vi "运维调试_采配水V1.vi"() -> ()   [LabVIEW 2016, in "PLC.lvlib"]
uses:
  PLC.lvlib
  <vilib>/Plasmionique/MB Master/MB_Master/MB_Master.lvclass
  <vilib>/Utility/miscctls.llb/LVPointTypeDef.ctl
  <vilib>/Plasmionique/MB Master/MB_Master_Serial/MB_Master_Serial.lvclass
  C:/Program Files (x86)/National Instruments/LabVIEW 2016/vi.lib/Plasmionique/MB Master/MB_Master/MB_Master.lvclass
  <vilib>/Instr/_visa.llb/VISA Configure Serial Port (Instr).vi
  <vilib>/Plasmionique/MB Master/MB Master.lvlib
panel:
  out "Registers":u16[](array[numeric])
  out "R118":i16 caption="多参数沉淀时间"
  in  "更新程序":bool
  out "当前启动泵号":u16(ring) items=["1号水样泵", "2号水样泵"]
  out "R113":i16 caption="储水时间设定"
  out "X2":bool caption="X1"
  out "采配水版本号":string
  out "R23":i16 caption="清洗频次计数"
  out "R112":i16 caption="清洗频次设定"
  out "R22":i16
  in  "Y15":bool
  out "R111":i16 caption="排液时间"
  out "通讯故障":bool
  out "R21":i16
  in  "Y14":bool
  out "R20":i16
  in  "Y13":bool
  in  "潜水泵工作模式":u16(ring) items=["泵1单泵单管路", "泵2单泵单管路", "潜水泵双泵双管路", "自吸泵双泵双管路"]
  out "X10":bool caption="废液报警"
  out "X9":bool caption="自来水检测"
  out "X8":bool caption="泵2过载报警"
  out "X7":bool caption="泵1过载报警"
  out "X6":bool caption="断电检测"
  out "X5":bool caption="开门检测"
  out "X4":bool caption="烟雾检测"
  out "X3":bool caption="漏水检测"
  out "X1":bool
  out "X0":bool caption="采样池液位开关"
  out "R109":i16 caption="配水时间"
  out "集成报警信息":string
  out "R108":i16 caption="自来水报警"
  out "R107":i16 caption="采水池液位报警设置"
  out "R106":i16 caption="进样超时设置"
  out "R105":i16 caption="二级清洗时间"
  out "R104":i16 caption="一级清洗时间"
  out "R103":i16 caption="外部管路清洗时间"
  out "R102":i16 caption="静置沉淀时间"
  out "R101":i16 caption="内部管路润洗时间"
  out "R100":i16 caption="外部管路润洗时间"
  out "R2":i16
  out "R1":i16
  out "多列列表框":i32(listbox)
  out "R19":i16
  in  "Y7":bool
  out "R18":i16
  in  "Y6":bool
  out "R17":i16
  in  "Y5":bool
  out "R16":i16
  in  "Y4":bool
  out "R15":i16
  in  "Y3":bool
  out "R14":i16
  in  "Y2":bool
  out "R13":i16
  in  "Y1":bool
  out "R12":i16
  in  "Y0":bool
  in  "返回":bool
  in  "参数设置":bool
  in  "单步启动":bool
  in  "启动":bool
  in  "停止":bool
  # "S"
  # "S"
  # "次"
  # "次"
  # "S"
  # "S"
  # "S"
  # "S"
  # "S"
  # "S"
  # "S"
  # "S"
  # "S"
  # "S"
  # "S"
  # "单步计时："
  # "s"
  # "流程计时："
  # "s"
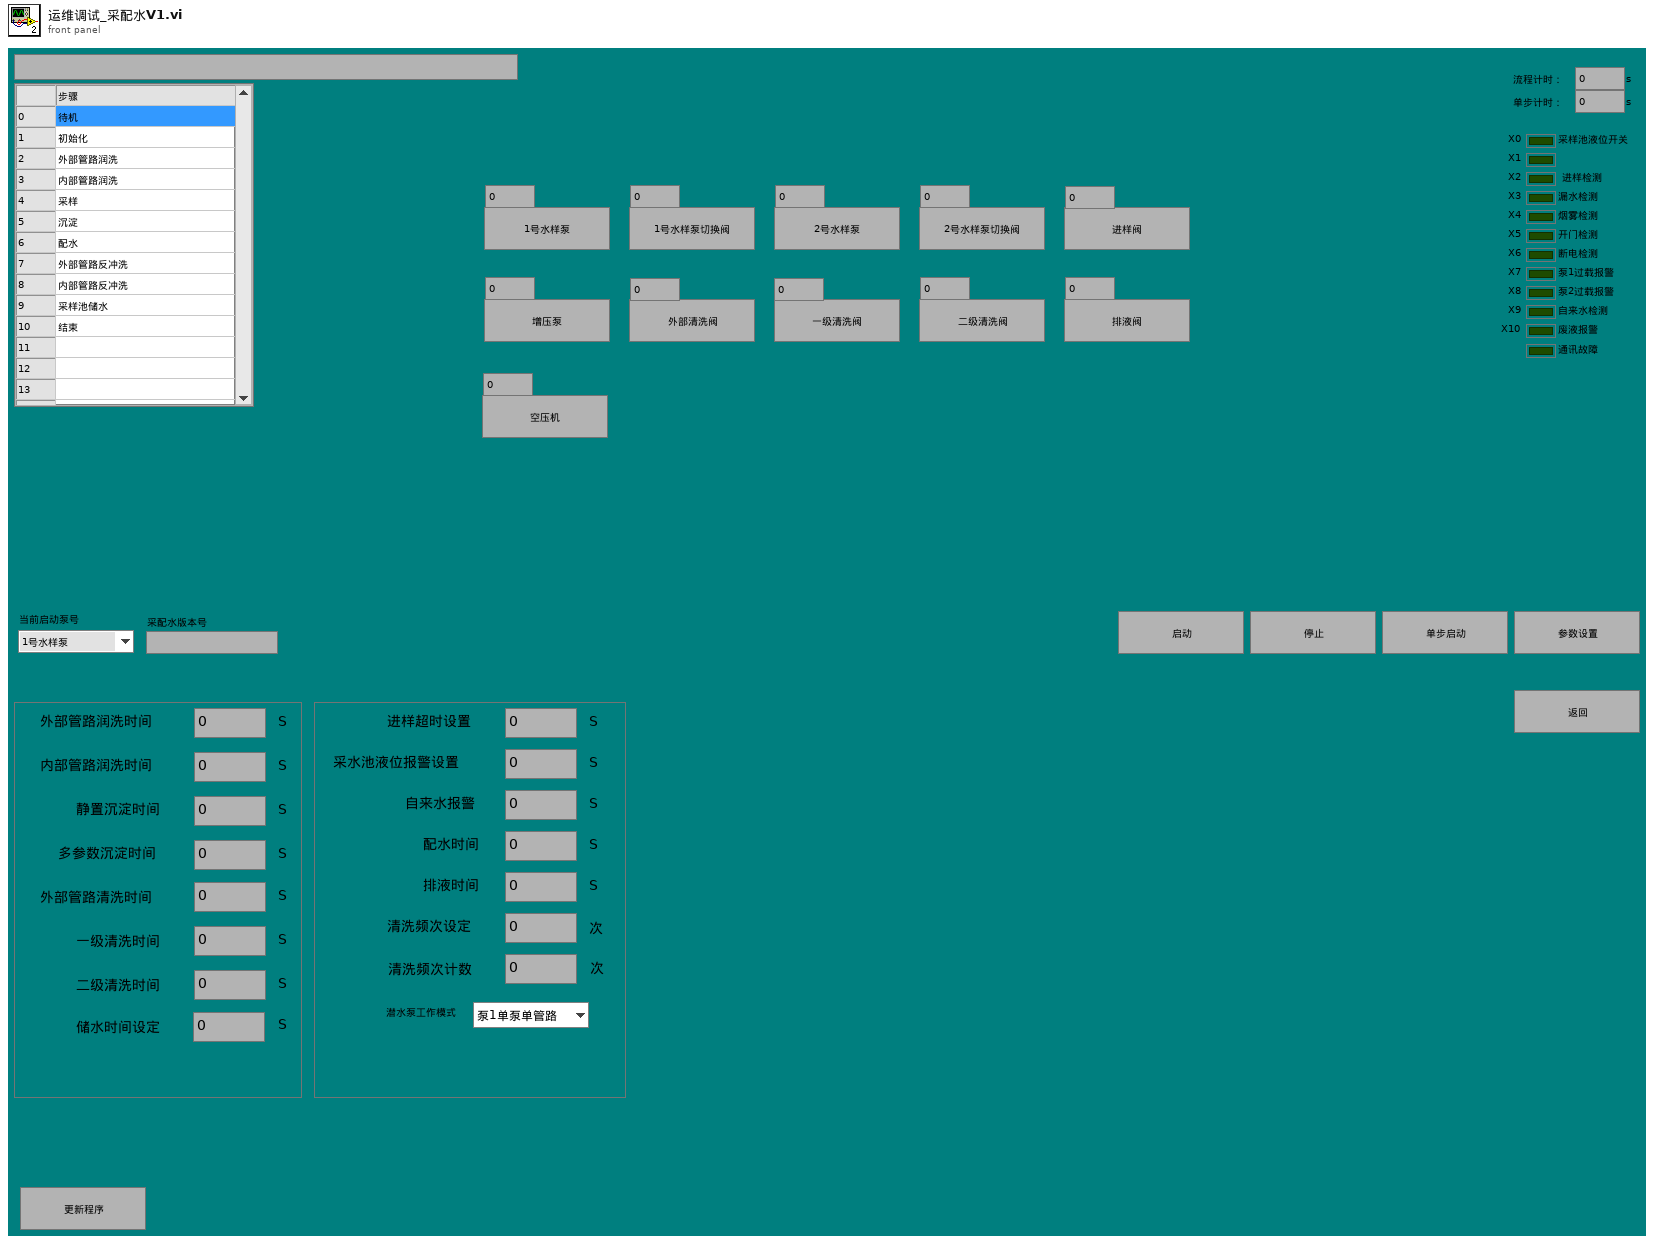
[diagram p1: front panel]
types:
  T1 = typedef "参数.ctl" = cluster{"测试模式":enum16{"水样测试", "平行样测试", "集成干预测试", "加标回收"}, "参数启用":T2}
  T2 = typedef "启动参数.ctl" = cluster{"氨氮":bool, "总磷":bool, "总氮":bool, "多参数":bool, "CODmn":bool, "CODCr":bool, "氟化物":bool, "超标留样启用":bool, "重金属":bool}
  T3 = typedef "LVPointTypeDef.ctl" = cluster{"Horizontal":i16, "Vertical":i16}
  T4 = cluster{"命令":string, "数据":cluster{"starting address":u16, "holding register value":u16}}
  T5 = cluster{"R0":i16, "R1":i16, "R2":i16, "R3":i16, "R4":i16, "R5":i16, "R6":i16, "R7":i16, "R8":i16, "R9":i16, "R10":i16, "R11":i16, "R12":i16, "R13":i16, "R14":i16, "R15":i16, "R16":i16, "R17":i16, "R18":i16, "R19":i16, "R20":i16, "R21":i16, "R22":i16, "R23":i16, "R24":i16, "R25":i16, "R26":i16, "R27":i16, "R28":i16, "R29":i16, "R30":i16, "R31":i16, "R32":i16, "R33":i16, "R34":i16, "R35":i16, "R36":i16, "R37":i16, "R38":i16, "R39":i16, "R40":i16, "R41":i16, "R42":i16, "R43":i16, "R44":i16, "R45":i16, "R46":i16, "R47":i16, "R48":i16, "R49":i16, "R50":i16, "R51":i16, "R52":i16, "R53":i16, "R54":i16, "R55":i16, "R56":i16, "R57":i16, "R58":i16, "R59":i16, "R60":i16, "R61":i16, "R62":i16, "R63":i16, "R64":i16, "R65":i16, "R66":i16, "R67":i16, "R68":i16, "R69":i16, "R70":i16, "R71":i16, "R72":i16, "R73":i16, "R74":i16, "R75":i16, "R76":i16, "R77":i16, "R78":i16, "R79":i16}
  T6 = cluster{"seconds since 1Jan1904":timestamp, "table输入":string, string, "table输入":string}
  T7 = cluster{"命令":string, cluster{"starting address":u16, "holding register value":u16}}
  T8 = cluster{"命令":string, "数据":cluster{"starting address":u16, "holding register values":u16[]}}
  T9 = cluster{"命令":string, "data":cluster{"starting address":u16, "coil values":bool[]}}
  T10 = cluster{"测试模式":enum16{"水样测试", "平行样测试", "集成干预测试", "加标回收"}, "参数启用":T2}
  T11 = cluster{"baud rate (bps)":u32, "stop bits":u16, "parity":u16, "flow control":u16, "timeout":u32, "retries":i32}
  T12 = cluster{"starting address":u16, "holding register values":u16[]}
  T13 = cluster{"starting address":u16, "holding register value":u16}
  T14 = cluster{"starting address":u16, "coil values":bool[]}
  T15 = cluster{"Registers[0]":u16, "Registers[1]":u16, "Registers[2]":u16, "Registers[3]":u16, "Registers[4]":u16, "Registers[5]":u16, "Registers[6]":u16, "Registers[7]":u16, "Registers[8]":u16, "Registers[9]":u16, "Registers[10]":u16, "Registers[11]":u16, "Registers[12]":u16, "Registers[13]":u16, "Registers[14]":u16, "Registers[15]":u16, "Registers[16]":u16, "Registers[17]":u16, "Registers[18]":u16, "Registers[19]":u16, "Registers[20]":u16, "Registers[21]":u16, "Registers[22]":u16, "Registers[23]":u16, "Registers[24]":u16, "Registers[25]":u16, "Registers[26]":u16, "Registers[27]":u16, "Registers[28]":u16, "Registers[29]":u16, "Registers[30]":u16, "Registers[31]":u16, "Registers[32]":u16, "Registers[33]":u16, "Registers[34]":u16, "Registers[35]":u16, "Registers[36]":u16, "Registers[37]":u16, "Registers[38]":u16, "Registers[39]":u16, "Registers[40]":u16, "Registers[41]":u16, "Registers[42]":u16, "Registers[43]":u16, "Registers[44]":u16, "Registers[45]":u16, "Registers[46]":u16, "Registers[47]":u16, "Registers[48]":u16, "Registers[49]":u16, "Registers[50]":u16, "Registers[51]":u16, "Registers[52]":u16, "Registers[53]":u16, "Registers[54]":u16, "Registers[55]":u16, "Registers[56]":u16, "Registers[57]":u16, "Registers[58]":u16, "Registers[59]":u16, "Registers[60]":u16, "Registers[61]":u16, "Registers[62]":u16, "Registers[63]":u16, "Registers[64]":u16, "Registers[65]":u16, "Registers[66]":u16, "Registers[67]":u16, "Registers[68]":u16, "Registers[69]":u16, "Registers[70]":u16, "Registers[71]":u16, "Registers[72]":u16, "Registers[73]":u16, "Registers[74]":u16, "Registers[75]":u16, "Registers[76]":u16, "Registers[77]":u16, "Registers[78]":u16, "Registers[79]":u16}
  T16 = cluster{"Registers[0]":u16, "Registers[1]":u16, "Registers[2]":u16, "Registers[3]":u16, "Registers[4]":u16, "Registers[5]":u16}
  T17 = cluster{"Registers[0]":u16, "Registers[1]":u16, "Registers[2]":u16, "Registers[3]":u16, "Registers[4]":u16, "Registers[5]":u16, "Registers[6]":u16, "Registers[7]":u16, "Registers[8]":u16, "Registers[9]":u16, "Registers[10]":u16, "Registers[11]":u16, "Registers[12]":u16, "Registers[13]":u16, "Registers[14]":u16, "Registers[15]":u16, "Registers[16]":u16, "Registers[17]":u16, "Registers[18]":u16, "Registers[19]":u16, "Registers[20]":u16, "Registers[21]":u16, "Registers[22]":u16, "Registers[23]":u16, "Registers[24]":u16, "Registers[25]":u16, "Registers[26]":u16, "Registers[27]":u16, "Registers[28]":u16, "Registers[29]":u16, "Registers[30]":u16, "Registers[31]":u16, "Registers[32]":u16, "Registers[33]":u16}
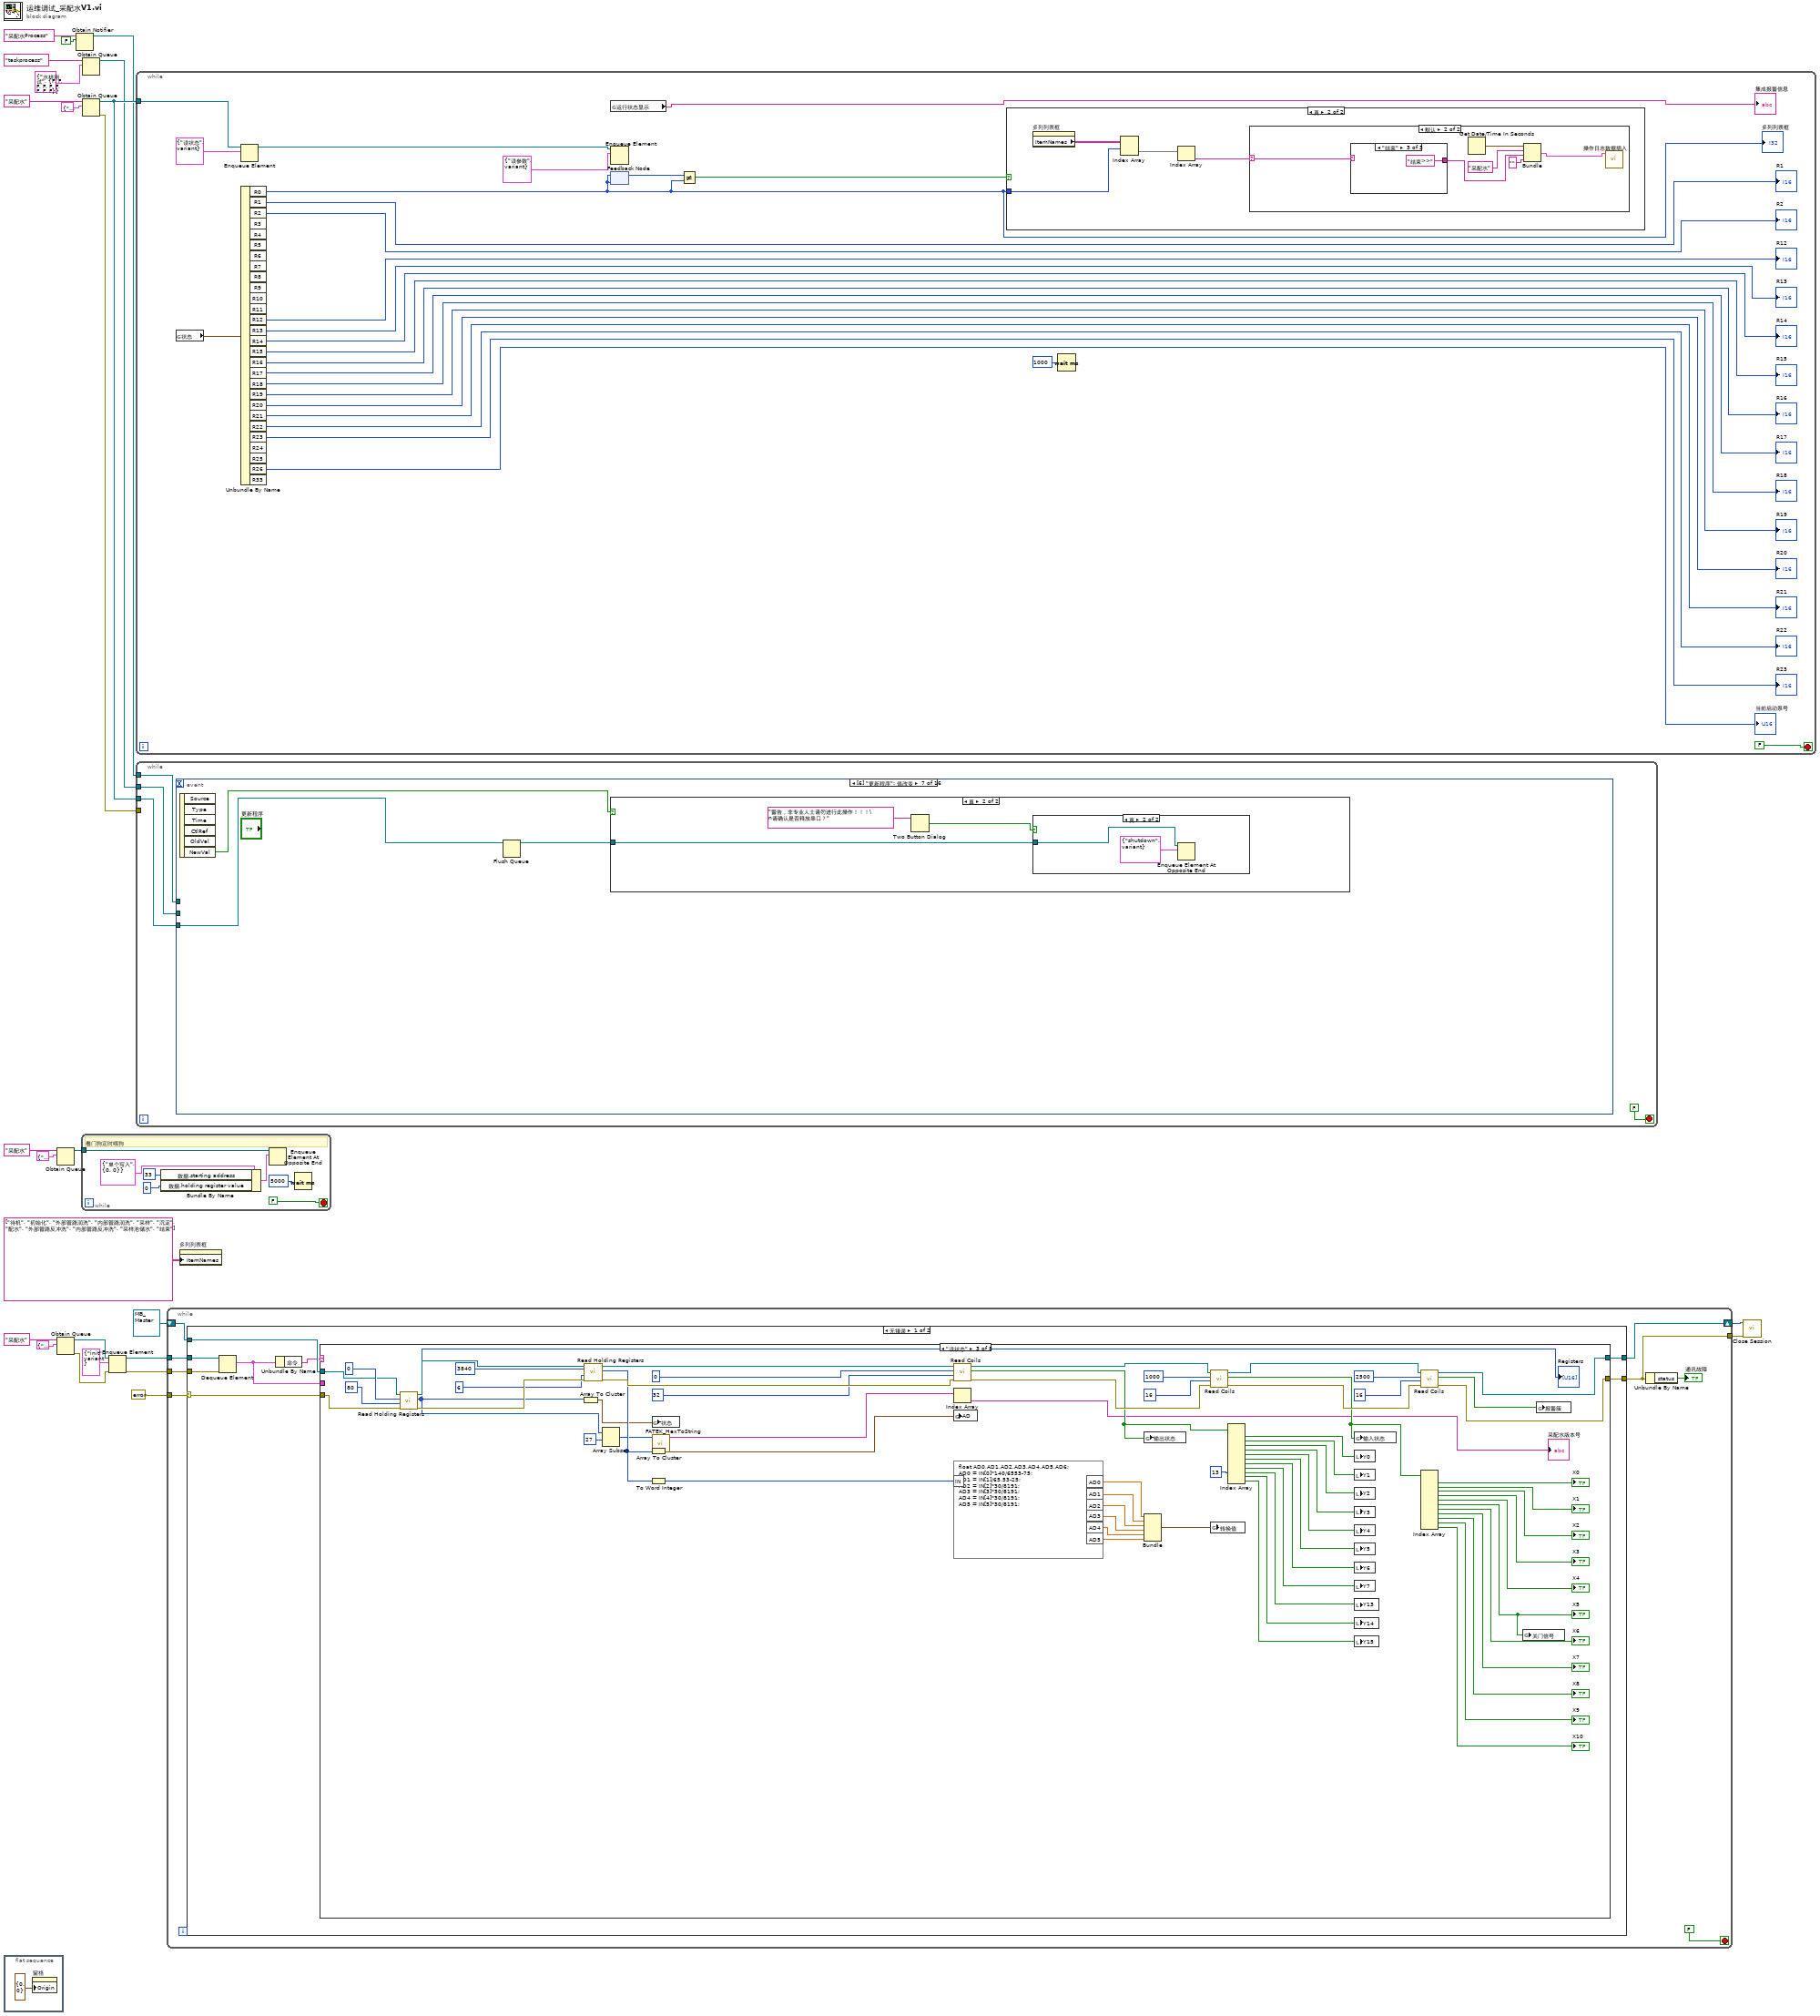
[diagram p0: block diagram]
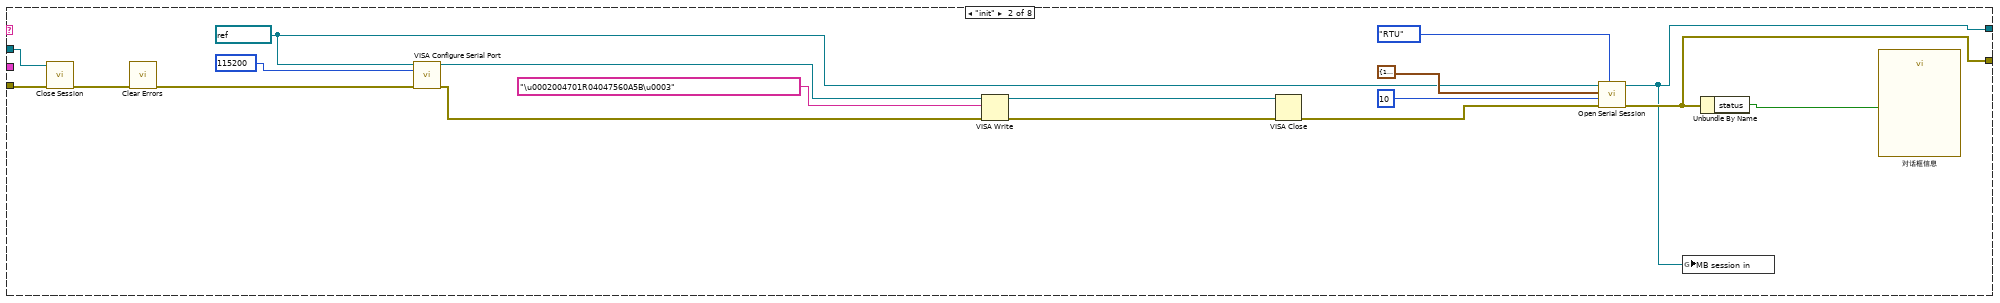
[diagram p3: hidden frame]
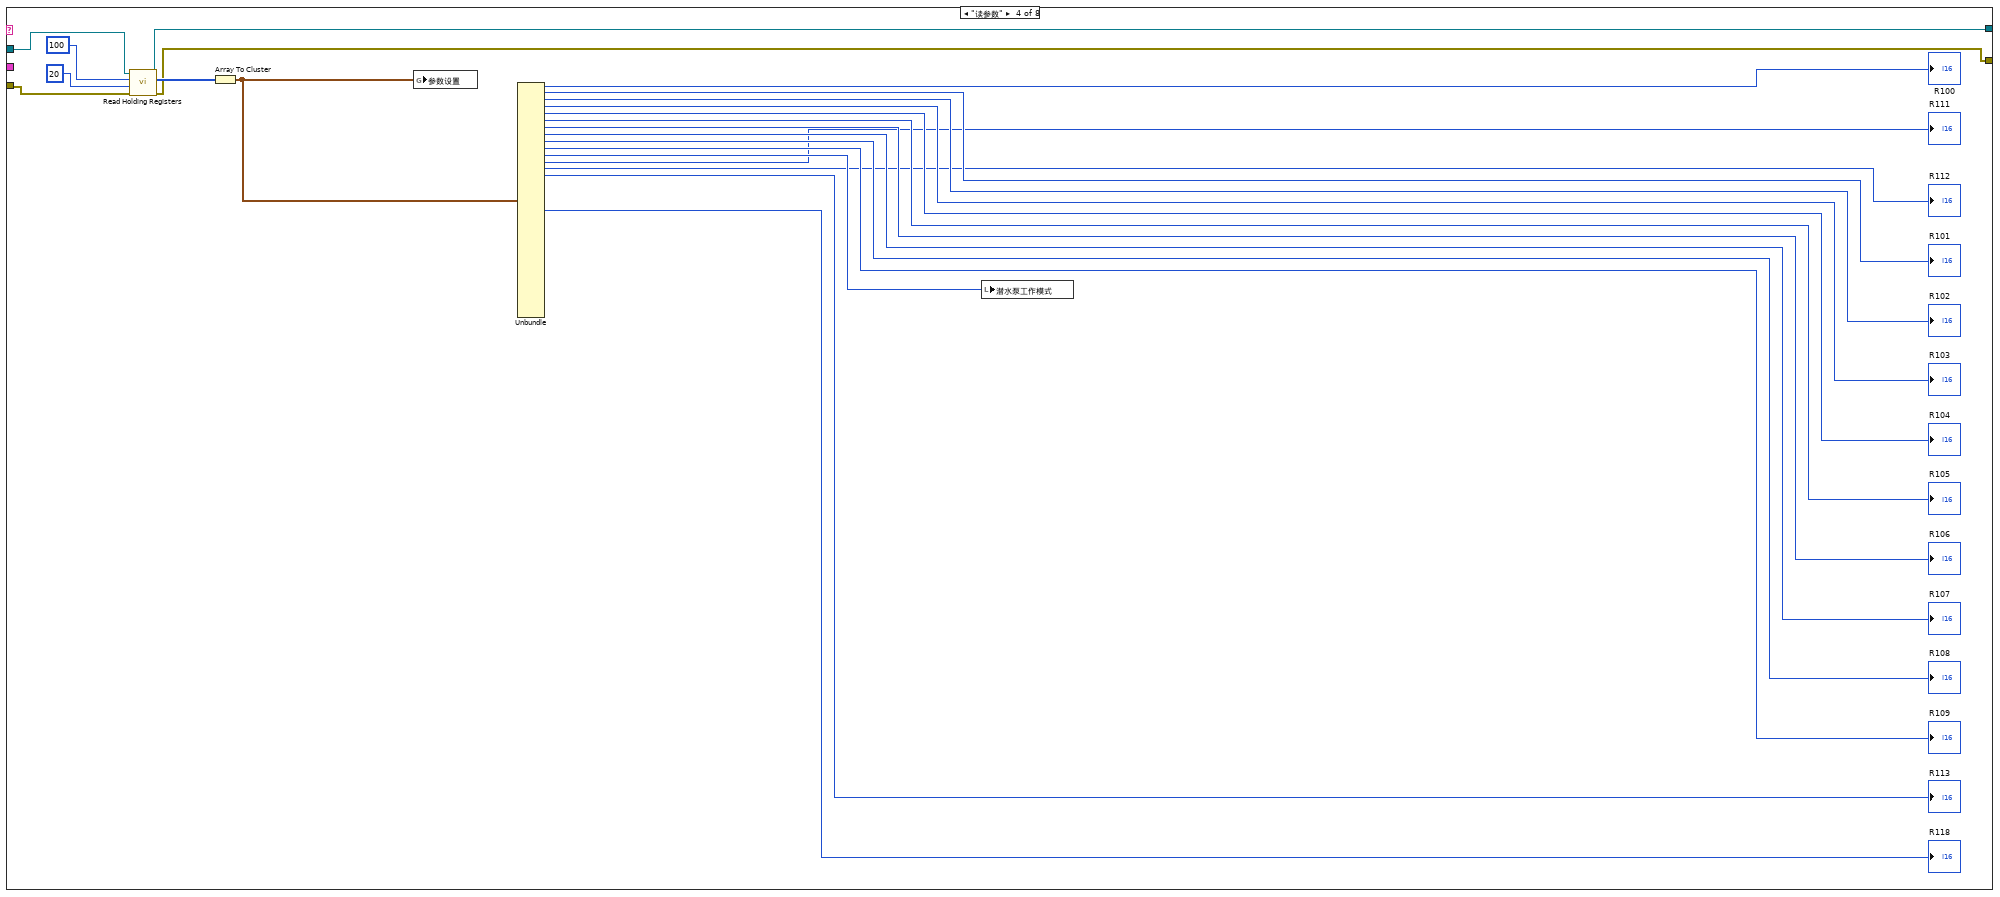
[diagram p4: hidden frame]
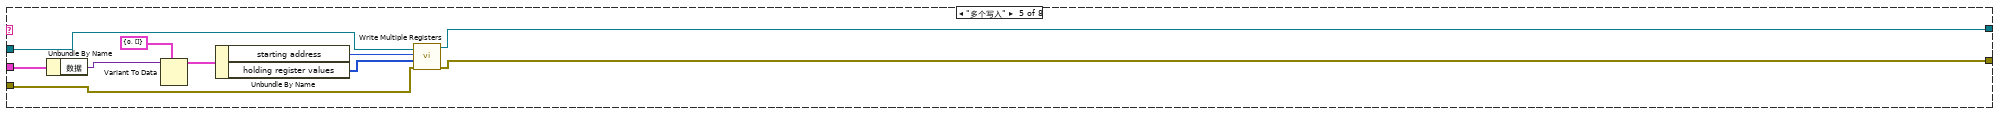
[diagram p5: hidden frame]
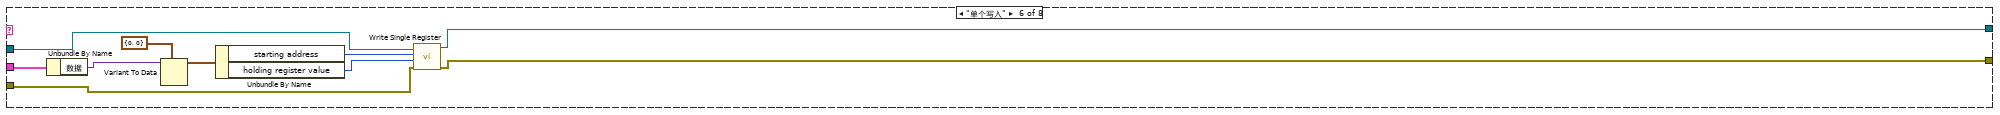
[diagram p6: hidden frame]
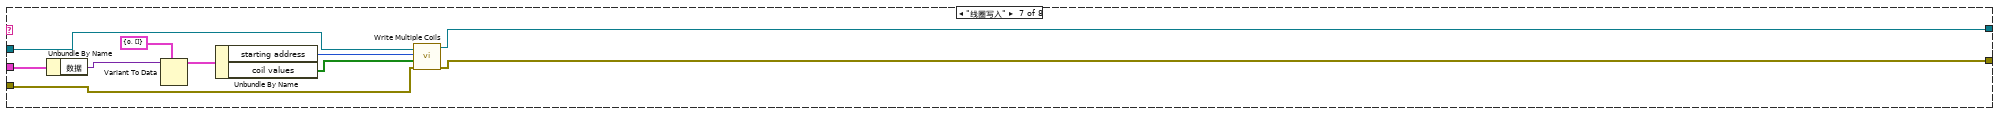
[diagram p7: hidden frame]
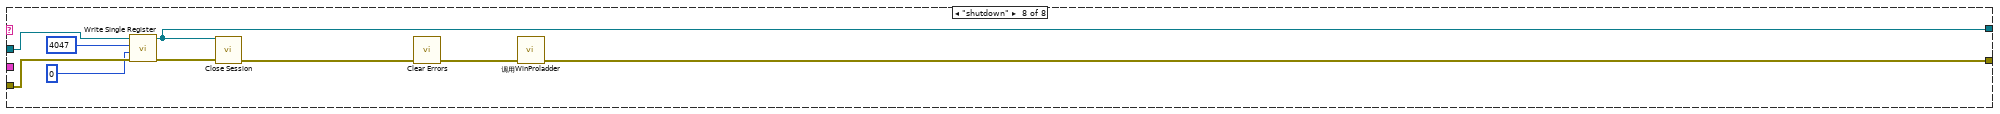
[diagram p8: hidden frame]
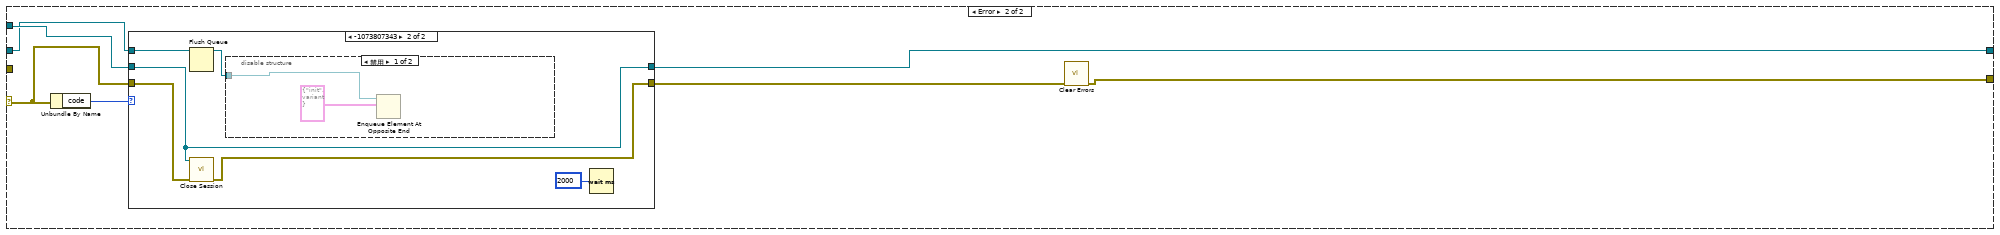
[diagram p9: hidden frame]
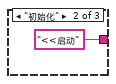
[diagram p15: hidden frame]
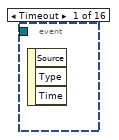
[diagram p16: hidden frame]
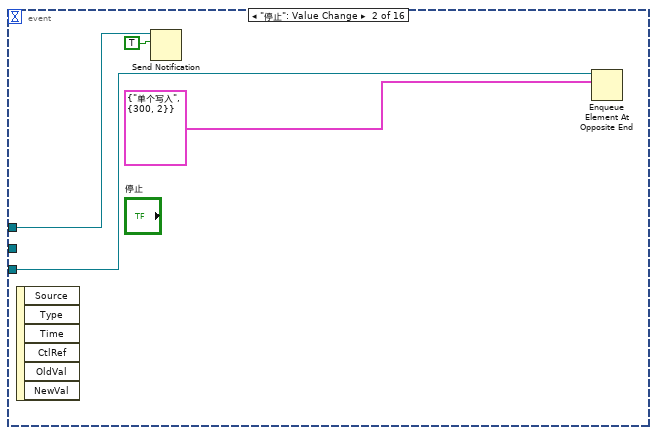
[diagram p17: hidden frame]
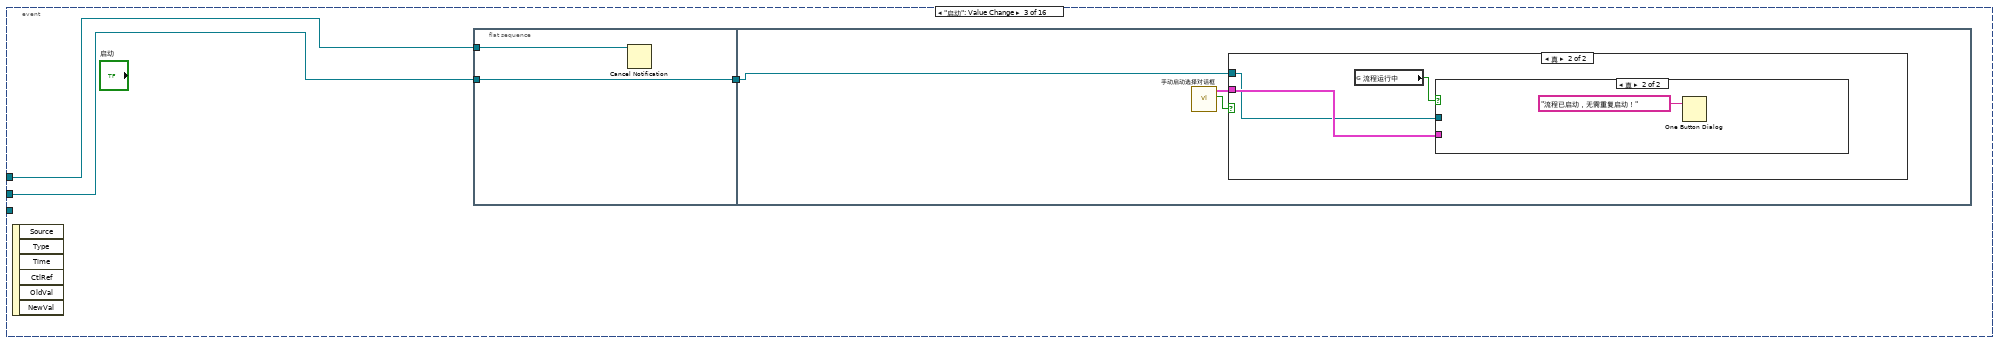
[diagram p18: hidden frame]
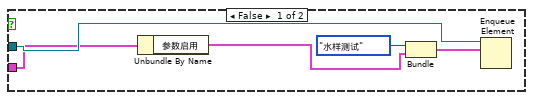
[diagram p20: hidden frame]
diagram:
  n1 = flat-sequence {
    frame #0 {
      n2 = property on="窗格" class="Pane"("Origin"=T3 {"Horizontal"=0, "Vertical"=0} ("原点")) -> ()  [unwired: 2 in, 2 out]
    }
  }
  n3 = Obtain Queue(name (unnamed)="采配水" ("名称（未命名）"), element data type=cluster{"命令":string, "数据":variant} {"命令"="", "数据"=variant}) -> (queue out=w4:refnum<queue>)  [unwired: 3 in, 2 out]
  n4 = Obtain Queue(name (unnamed)="采配水" ("名称（未命名）"), element data type=cluster{"命令":string, "数据":variant} {"命令"="", "数据"=variant}) -> (queue out=w15:refnum<queue>, error out=w14:errorcluster)  [unwired: 3 in, 1 out]
  n5 = Obtain Notifier(name (unnamed)="采配水Process" ("名称（未命名）"), notification data type=FALSE) -> (notifier out=w18:refnum<notifier>)  [unwired: 2 in, 2 out]
  n6 = while {
    tunnel: w4 -> [w29]
    stop <- FALSE stop-if-true
    # "看门狗定时喂狗"
    n7 = Bundle By Name(cluster=T4 {"命令"="单个写入", "数据"={"starting address"=0, "holding register value"=0}} ("元素"), "数据.starting address"=u16 33, "数据.holding register value"=u16 0) -> (w30:T4)
    n8 = Enqueue Element At Opposite End(queue=w29, element=w30) -> ()  [unwired: 2 in, 3 out]
    n9 = Wait (ms)(milliseconds to wait=u32 5000 ("等待时间（毫秒）")) -> ()  [unwired: 1 out]
  }
  n10 = Obtain Queue(name (unnamed)="taskprocess" ("名称（未命名）"), element data type=T1 {"测试模式"=enum."水样测试", "参数启用"={"氨氮"=FALSE, "总磷"=FALSE, "总氮"=FALSE, "多参数"=FALSE, "CODmn"=FALSE, "CODCr"=FALSE, "氟化物"=FALSE, "超标留样启用"=FALSE, "重金属"=FALSE}} ("参数")) -> (queue out=w2:refnum<queue>)  [unwired: 3 in, 2 out]
  n11 = Obtain Queue(name (unnamed)="采配水" ("名称（未命名）"), element data type=cluster{"命令":string, "数据":variant} {"命令"="", "数据"=variant}) -> (queue out=w22:refnum<queue>, error out=w23:errorcluster)  [unwired: 3 in, 1 out]
  n12 = Enqueue Element(queue=w15, element=cluster{"命令":string, "数据":variant} {"命令"="init", "数据"=variant} ("元素"), error in (no error)=w14) -> (queue out=w10:refnum<queue>, error out=w12:errorcluster)  [unwired: 1 in, 1 out]
  n13 = while {
    tunnel: w22 -> [w58]
    stop <- FALSE stop-if-true
    n14 = global read "采配水全局变量.vi" "状态"() -> (w56:T5)
    n15 = Enqueue Element(queue=w58, element=cluster{"命令":string, "数据":variant} {"命令"="读状态", "数据"=variant} ("元素")) -> (queue out=w41:refnum<queue>)  [unwired: 2 in, 2 out]
    n16 = Unbundle By Name(w56) -> ("R0"=w39:i16, "R1"=→"R1":i16, "R2"=→"R2":i16, "R12"=→"R12":i16, "R13"=→"R13":i16, "R14"=→"R14":i16, "R15"=→"R15":i16, "R16"=→"R16":i16, "R17"=→"R17":i16, "R18"=→"R18":i16, "R19"=→"R19":i16, "R20"=→"R20":i16, "R21"=→"R21":i16, "R22"=→"R22":i16, "R23"=→"R23":i16, "R26"=→"当前启动泵号":i16)  [unwired: 12 out]
    "多列列表框" <- w39
    n17 = global read "采配水全局变量.vi" "运行状态显示"() -> (→"集成报警信息":string)
    n18 = Enqueue Element(queue=w41, element=cluster{"命令":string, "数据":variant} {"命令"="读参数", "数据"=variant} ("元素")) -> ()  [unwired: 2 in, 3 out]
    n19 = feedback-in #1(w39) -> ()
    n20 = feedback #1(w39) -> (w40:i16)
    n21 = Not Equal?(x=w40, y=w39) -> (x != y?=w45:bool)
    n22 = case shown="真" w45 {
      tunnel: w39 -> [_ w62]
      frame False {
      }
      frame True {
        n23 = property on="多列列表框" class="MCListbox (严格)"() -> ("ItemNames"=w63:string[][])  [unwired: 2 in, 2 out]
        n24 = Index Array(array=w63, index (row)=w62) -> (element=w61:string[])  [unwired: 1 in]
        n25 = Index Array(array=w61) -> (element=w60:string)  [unwired: 1 in]
        n26 = case shown="默认" w60 {
          selector: w60 -> [_ w64]
          frame "待机" {
          }
          frame Default {
            n27 = case shown="\"结束\"" w64 {
              selector: w64 -> [w70 _ _]
              tunnel: [w70 "<<启动" "结束>>"] -> w66
              frame Default {
              }
              frame "初始化" {
              }
              frame "结束" {
              }
            }
            n28 = Get Date/Time In Seconds() -> (seconds since 1Jan1904=w69:timestamp)
            n29 = Bundle("seconds since 1Jan1904"=w69, "table输入"="采配水", w66, "table输入"="") -> (w65:T6)  [unwired: 1 in]
            n30 = call "操作日志数据插入.vi"("data"=w65) -> ()  [unwired: 9 in, 1 out]
          }
        }
      }
    }
    n31 = Wait (ms)(milliseconds to wait=u32 1000 ("等待时间（毫秒）")) -> ()  [unwired: 1 out]
  }
  n32 = while {
    tunnel: w22 -> [w75]
    tunnel: w23 -> [_]
    tunnel: w18 -> [w74]
    tunnel: w2 -> [w73]
    stop <- FALSE stop-if-true
    n33 = event shown="[6] \"更新程序\": 值改变" {
      selector: _ -> [_ _ _ _ _ _ _ _ _ _ _ _ _ _ _ _]
      dyn-events: _ -> [_ _ _ _ _ _ _ _ _ _ _ _ _ _ _ _]
      timeout: _ -> [_ _ _ _ _ _ _ _ _ _ _ _ _ _ _ _]
      tunnel: w75 -> [_ w79 _ w101 w120 w123 w129 w140 _ _ _ _ w168 w170 w175 w180]
      tunnel: w74 -> [_ w78 w83 _ _ _ _ _ _ _ _ _ _ _ _ _]
      tunnel: w73 -> [_ _ w81 _ _ _ _ _ _ _ _ _ _ _ _ _]
      event Timeout {
        n34 = event-data() -> ()  [unwired: 1 in, 3 out]
      }
      event "停止": Value Change {
        n35 = event-data() -> ()  [unwired: 1 in, 6 out]
        n36 = Send Notification(notification=TRUE ("通知"), notifier=w78) -> ()  [unwired: 1 in, 2 out]
        n37 = Enqueue Element At Opposite End(queue=w79, element=T7 {"命令"="单个写入", {"starting address"=300, "holding register value"=2}} ("元素")) -> ()  [unwired: 2 in, 3 out]
      }
      event "启动": Value Change {
        n38 = event-data() -> ()  [unwired: 1 in, 6 out]
        n39 = flat-sequence {
          tunnel: w83 -> [w85]
          tunnel: [w84] -> w82
          tunnel: w81 -> [w84]
          tunnel: w82 -> [w86]
          frame #0 {
            n40 = Cancel Notification(0:w85) -> ()  [unwired: 1 in, 3 out]
          }
          frame #1 {
            n41 = call "手动启动选择对话框.vi"() -> ("确定"=w87:bool, "输出簇"=w88:cluster{"参数启用":T2})  [unwired: 10 in]
            n42 = case shown="真" w87 {
              tunnel: w88 -> [_ w91]
              tunnel: w86 -> [_ w90]
              frame False {
              }
              frame True {
                n43 = global read "采配水全局变量.vi" "流程运行中"() -> (w89:bool)
                n44 = case shown="真" w89 {
                  tunnel: w91 -> [w94 _]
                  tunnel: w90 -> [w96 _]
                  frame False {
                    n45 = Unbundle By Name(w94) -> ("参数启用"=w93:T2)
                    n46 = Bundle("测试模式"=enum16{"水样测试", "平行样测试", "集成干预测试", "加标回收"}."水样测试", "参数启用"=w93) -> (w92:T10)  [unwired: 1 in]
                    n47 = Enqueue Element(queue=w96, element=w92) -> ()  [unwired: 2 in, 3 out]
                  }
                  frame True {
                    n48 = One Button Dialog(message="流程已启动，无需重复启动！" ("消息")) -> ()  [unwired: 1 in, 1 out]
                  }
                }
              }
            }
          }
        }
      }
      event "单步启动": Value Change {
        n49 = event-data() -> ()  [unwired: 1 in, 6 out]
        n50 = call "单步启动对话框.vi"() -> ("单步启动步骤输出"=w98:u16)  [unwired: 11 in]
        n51 = Bundle By Name(cluster=T4 {"命令"="单个写入", "数据"={"starting address"=301, "holding register value"=0}} ("元素"), "数据.holding register value"=w98) -> (w99:T4)
        n52 = Enqueue Element At Opposite End(queue=w101, element=w99) -> ()  [unwired: 2 in, 3 out]
      }
      event "R100", "R101", "R102", "R103", "R104", "R105", "R106", "R107", "R108", "R109", "潜水泵工作模式", "R111", "R112", "R113": Value Change {
        n53 = event-data() -> ()  [unwired: 1 in, 6 out]
        n54 = local read "R100"() -> (w115:i16)
        n55 = local read "R101"() -> (w114:i16)
        n56 = local read "R102"() -> (w113:i16)
        n57 = local read "R103"() -> (w112:i16)
        n58 = local read "R104"() -> (w111:i16)
        n59 = local read "R105"() -> (w110:i16)
        n60 = local read "R106"() -> (w109:i16)
        n61 = local read "R107"() -> (w108:i16)
        n62 = local read "R108"() -> (w107:i16)
        n63 = local read "R109"() -> (w106:i16)
        n64 = local read "R111"() -> (w104:i16)
        n65 = local read "R112"() -> (w103:i16)
        n66 = local read "R113"() -> (w102:i16)
        n67 = Build Array(w115, w114, w113, w112, w111, w110, w109, w108, w107, w106, "潜水泵工作模式", w104, w103, w102) -> (w116:u16[])
        n68 = Bundle By Name(cluster=T8 {"命令"="多个写入", "数据"={"starting address"=0, "holding register values"=[]}} ("元素"), "数据.starting address"=u16 100, "数据.holding register values"=w116) -> (w117:T8)
        n69 = Enqueue Element At Opposite End(queue=w120, element=w117) -> ()  [unwired: 2 in, 3 out]
      }
      event "R118": Value Change {
        n70 = event-data() -> ()  [unwired: 1 in, 6 out]
        n71 = local read "R118"() -> (w121:i16)
        n72 = Build Array(w121) -> (w122:i16[])
        n73 = Bundle By Name(cluster=T8 {"命令"="多个写入", "数据"={"starting address"=0, "holding register values"=[]}} ("元素"), "数据.starting address"=u16 118, "数据.holding register values"=w122) -> (w124:T8)
        n74 = Enqueue Element At Opposite End(queue=w123, element=w124) -> ()  [unwired: 2 in, 3 out]
      }
      event "更新程序": Value Change {
        n75 = event-data() -> ("NewVal"=w128:bool)  [unwired: 1 in, 5 out]
        n76 = Flush Queue(queue=w129) -> (queue out=w127:refnum<queue>)  [unwired: 1 in, 2 out]
        n77 = case shown="真" w128 {
          tunnel: w127 -> [w130 w134]
          frame False {
            n78 = Enqueue Element At Opposite End(queue=w130, element=cluster{"命令":string, "数据":variant} {"命令"="init", "数据"=variant} ("元素")) -> ()  [unwired: 2 in, 3 out]
          }
          frame True {
            n79 = Two Button Dialog(message="警告，非专业人士请勿进行此操作！！！\n请确认是否释放串口？" ("消息")) -> (T button?=w132:bool)  [unwired: 2 in]
            n80 = case shown="真" w132 {
              tunnel: w134 -> [_ w137]
              frame False {
                n81 = local write "更新程序"(FALSE ("下载模式")) -> ()
              }
              frame True {
                n82 = Enqueue Element At Opposite End(queue=w137, element=cluster{"命令":string, "数据":variant} {"命令"="shutdown", "数据"=variant} ("元素")) -> ()  [unwired: 2 in, 3 out]
              }
            }
          }
        }
      }
      event "R23": Value Change {
        n83 = event-data() -> ()  [unwired: 1 in, 6 out]
        n84 = local read "R23"() -> (w139:i16)
        n85 = Build Array(w139) -> (w138:i16[])
        n86 = Bundle By Name(cluster=T8 {"命令"="多个写入", "数据"={"starting address"=0, "holding register values"=[]}} ("元素"), "数据.starting address"=u16 23, "数据.holding register values"=w138) -> (w141:T8)
        n87 = Enqueue Element At Opposite End(queue=w140, element=w141) -> ()  [unwired: 2 in, 3 out]
      }
      event "R23": Mouse Down {
        n88 = event-data() -> ("CtlRef"=w146:refnum<vi>)  [unwired: 1 in, 7 out]
        n89 = Two Button Dialog(message="请确认是否更改，更改后将影响实际清洗频次" ("消息")) -> (T button?=w145:bool)  [unwired: 2 in]
        n90 = case shown="真" w145 {
          tunnel: w146 -> [_ w147]
          frame False {
          }
          frame True {
            n91 = property class="DigNum (严格)"(reference=w147) -> (reference out=w149:refnum<vi>, "Value"=w150:i16)  [unwired: 1 in, 1 out]
            n92 = call "数字键盘.vi"("OldNumber"=w150) -> ("NewNumber"=w148:sgl)
            n93 = property class="DigNum (严格)"(reference=w149, "Val(Sgnl)"=w148) -> ()  [unwired: 1 in, 2 out]
          }
        }
      }
      event "R100", "R101", "R102", "R103", "R104", "R105", "R106", "R107", "R108", "R109", "R111", "R112", "R113", "R118": Mouse Down {
        n94 = event-data() -> ("CtlRef"=w154:refnum<vi>)  [unwired: 1 in, 7 out]
        n95 = property class="DigNum (严格)"(reference=w154) -> (reference out=w152:refnum<vi>, "Value"=w153:i16)  [unwired: 1 in, 1 out]
        n96 = call "数字键盘.vi"("OldNumber"=w153) -> ("NewNumber"=w151:sgl)
        n97 = property class="DigNum (严格)"(reference=w152, "Val(Sgnl)"=w151) -> ()  [unwired: 1 in, 2 out]
      }
      event "参数设置": Value Change {
        n98 = event-data() -> ()  [unwired: 1 in, 6 out]
        n99 = property on="窗格" class="Pane"("Origin"=T3 {"Horizontal"=0, "Vertical"=628} ("原点")) -> ()  [unwired: 2 in, 2 out]
      }
      event "返回": Value Change {
        n100 = event-data() -> ()  [unwired: 1 in, 6 out]
        n101 = property on="窗格" class="Pane"("Origin"=T3 {"Horizontal"=0, "Vertical"=0} ("原点")) -> ()  [unwired: 2 in, 2 out]
      }
      event "Y0", "Y1", "Y2", "Y3", "Y4", "Y5", "Y6", "Y7": Value Change {
        n102 = event-data() -> ()  [unwired: 1 in, 6 out]
        n103 = Build Array("Y0", "Y1", "Y2", "Y3", "Y4", "Y5", "Y6", "Y7") -> (w157:bool[])
        n104 = Bundle By Name(cluster=T9 {"命令"="线圈写入", "data"={"starting address"=2400, "coil values"=[]}} ("元素"), "data.coil values"=w157) -> (w158:T9)
        n105 = Enqueue Element(queue=w168, element=w158) -> ()  [unwired: 2 in, 3 out]
      }
      event "Y13": Value Change {
        n106 = event-data() -> ()  [unwired: 1 in, 6 out]
        n107 = Build Array("Y13") -> (w171:bool[])
        n108 = Bundle By Name(cluster=T9 {"命令"="线圈写入", "data"={"starting address"=2413, "coil values"=[]}} ("元素"), "data.coil values"=w171) -> (w172:T9)
        n109 = Enqueue Element(queue=w170, element=w172) -> ()  [unwired: 2 in, 3 out]
      }
      event "Y14": Value Change {
        n110 = event-data() -> ()  [unwired: 1 in, 6 out]
        n111 = Build Array("Y14") -> (w176:bool[])
        n112 = Bundle By Name(cluster=T9 {"命令"="线圈写入", "data"={"starting address"=2414, "coil values"=[]}} ("元素"), "data.coil values"=w176) -> (w177:T9)
        n113 = Enqueue Element(queue=w175, element=w177) -> ()  [unwired: 2 in, 3 out]
      }
      event "Y15": Value Change {
        n114 = event-data() -> ()  [unwired: 1 in, 6 out]
        n115 = Build Array("Y15") -> (w181:bool[])
        n116 = Bundle By Name(cluster=T9 {"命令"="线圈写入", "data"={"starting address"=2415, "coil values"=[]}} ("元素"), "data.coil values"=w181) -> (w182:T9)
        n117 = Enqueue Element(queue=w180, element=w182) -> ()  [unwired: 2 in, 3 out]
      }
    }
  }
  n118 = while {
    tunnel: w10 -> [w188]
    tunnel: w12 -> [w187]
    shift-right: [w191] -> w7
    shift-left: refnum<class "MB_Master.lvclass"> refnum ("MB session in") -> [w190]
    tunnel: errorcluster {"status"=FALSE, "code"=0, "source"=""} ("error out") -> [w189]
    tunnel: [w186] -> w8
    stop <- FALSE stop-if-true
    n119 = case shown="无错误" w189 {
      selector: w189 -> [w196 w350]
      tunnel: [w199 w349] -> w191
      tunnel: w190 -> [w198 w351]
      tunnel: [w197 w347] -> w186
      tunnel: w188 -> [w194 w346]
      tunnel: w187 -> [w193 _]
      frame No Error {
        n120 = Dequeue Element(queue=w194, error in (no error)=w193) -> (element=w192:cluster{"命令":string, "数据":variant})  [unwired: 1 in, 3 out]
        n121 = Unbundle By Name(w192) -> ("命令"=w195:string)
        n122 = case shown="\"读状态\"" w195 {
          tunnel: [w201 w202 w235 w301 w313 w323 w333 w342] -> w199
          tunnel: w198 -> [w201 w216 w272 w306 w316 w326 w336 w345]
          tunnel: [w200 w215 w234 w300 w314 w324 w334 w337] -> w197
          tunnel: w196 -> [w200 w218 w275 w305 w315 w325 w335 w343]
          tunnel: w192 -> [_ _ _ _ w312 w322 w332 _]
          frame "idle", Default {
          }
          frame "init" {
            w207 = refnum<visa-resource-name> "COM3" ("VISA resource name")
            n123 = call-dynamic "Close Session.vi"("error in (no error)"=w218, "MB session in"=w216) -> ("error out"=w217:errorcluster)  [unwired: 9 in]
            n124 = call <vilib>:"Clear Errors.vi"("error in (no error)"=w217) -> ("error out"=w205:errorcluster)  [unwired: 5 in, 1 out]
            n125 = call-poly "VISA Configure Serial Port"("VISA resource name"=w207, "baud rate (9600)"=u32 115200, "error in (no error)"=w205) -> ("VISA resource name out"=w209:refnum<visa-resource-name>, "error out"=w211:errorcluster)  [unwired: 11 in]
            n126 = VISA Write(VISA resource name=w209, write buffer="\u0002004701R04047560A5B\u0003" ("写入缓冲区"), error in (no error)=w211) -> (VISA resource name out=w208:refnum<visa-resource-name>, error out=w210:errorcluster)  [unwired: 1 out]
            n127 = VISA Close(VISA resource name=w208, error in (no error)=w210) -> (error out=w204:errorcluster)
            n128 = call <vilib>:"Open Serial Session.vi"("Mode (RTU)"=enum16{"RTU", "ASCII"}."RTU", "Error in"=w204, "Slave ID"=u8 10, "Serial Config"=T11 {"baud rate (bps)"=115200, "stop bits"=10, "parity"=0, "flow control"=0, "timeout"=500, "retries"=1}, "VISA Resource"=w207) -> ("Error out"=w215:errorcluster, "MB_Serial session"=w202:refnum<class "MB_Master_Serial.lvclass">)  [unwired: 5 in]
            n129 = global write "采配水全局变量.vi" "MB session in"(w202) -> ()
            n130 = Unbundle By Name(w215) -> ("status"=w219:bool)
            n131 = call "对话框信息"("Enable"=w219) -> ()  [unwired: 9 in, 2 out]
          }
          frame "读状态" {
            n132 = call <vilib>:"Read Holding Registers.vi"("error in (no error)"=w275, "quantity"=u16 80 ("number of holding registers"), "starting address"=u16 0, "MB session in"=w272) -> ("error out"=w270:errorcluster, "Registers"=w232:u16[], "MB session out"=w271:refnum<class "MB_Master.lvclass">)  [unwired: 5 in]
            "Registers" <- w232
            n133 = Array To Cluster(array=w232) -> (cluster=w233:T15)
            n134 = call <vilib>:"Read Holding Registers.vi"("error in (no error)"=w270, "quantity"=u16 6 ("number of holding registers"), "starting address"=u16 3840, "MB session in"=w271) -> ("error out"=w266:errorcluster, "Registers"=w245:u16[], "MB session out"=w267:refnum<class "MB_Master.lvclass">)  [unwired: 5 in]
            n135 = Array Subset(array=w232, index=27 ("索引")) -> (w242:u16[])  [unwired: 1 in]
            n136 = Array To Cluster(array=w245) -> (cluster=w283:T16)
            n137 = To Word Integer(number=w245) -> (16bit integer=w244:i16[])
            n138 = global write "采配水全局变量.vi" "状态"(w233) -> ()
            n139 = call "FATEK_HexToString.vi"("数组"=w242) -> ("STRING"=w241:string[])  [unwired: 10 in]
            n140 = call <vilib>:"Read Coils.vi"("error in (no error)"=w266, "quantity"=u16 32 ("number of coils"), "starting address"=u16 0, "MB session in"=w267) -> ("error out"=w262:errorcluster, "Coils"=w248:bool[], "MB session out"=w263:refnum<class "MB_Master.lvclass">)  [unwired: 5 in]
            n141 = Index Array(array=w241) -> (element=→"采配水版本号":string)  [unwired: 1 in]
            n142 = global write "采配水全局变量.vi" "AD"(w283) -> ()
            n143 = formula code="float AD0,AD1,AD2,AD3,AD4,AD5,AD6;\nAD0 = IN[0]*140/6553-75;\nAD1 = IN[1]/65.53-25;\nAD2 = IN[2]*30/8191;\nAD3 = IN[3]*30/8191;\nAD4 = IN[4]*30/8191;\nAD5 = IN[5]*30/8191;"("IN"=w244) -> ("AD0"=w281:dbl, "AD1"=w280:dbl, "AD2"=w279:dbl, "AD3"=w278:dbl, "AD4"=w277:dbl, "AD5"=w276:dbl)
            n144 = global write "采配水全局变量.vi" "输出状态"(w248) -> ()
            n145 = Bundle(w281, w280, w279, w278, w277, w276) -> (w282:cluster{dbl, dbl, dbl, dbl, dbl, dbl})  [unwired: 1 in]
            n146 = call <vilib>:"Read Coils.vi"("error in (no error)"=w262, "quantity"=u16 16 ("number of coils"), "starting address"=u16 1000, "MB session in"=w263) -> ("error out"=w258:errorcluster, "Coils"=w254:bool[], "MB session out"=w259:refnum<class "MB_Master.lvclass">)  [unwired: 5 in]
            n147 = global write "采配水全局变量.vi" "转换值"(w282) -> ()
            n148 = Index Array(array=w248, index #9=13 ("索引")) -> (element #1=w231:bool, element #2=w239:bool, element #3=w230:bool, element #4=w229:bool, element #5=w228:bool, element #6=w227:bool, element #7=w226:bool, element #8=w225:bool, element #9=w223:bool, element #10=w222:bool, element #11=w221:bool)  [unwired: 10 in]
            n149 = global write "采配水全局变量.vi" "输入状态"(w254) -> ()
            n150 = local write "Y0"(w231) -> ()
            n151 = local write "Y1"(w239) -> ()
            n152 = local write "Y2"(w230) -> ()
            n153 = local write "Y3"(w229) -> ()
            n154 = local write "Y4"(w228) -> ()
            n155 = local write "Y5"(w227) -> ()
            n156 = local write "Y6"(w226) -> ()
            n157 = local write "Y7"(w225) -> ()
            n158 = local write "Y13"(w223) -> ()
            n159 = local write "Y14"(w222) -> ()
            n160 = local write "Y15"(w221) -> ()
            n161 = call <vilib>:"Read Coils.vi"("error in (no error)"=w258, "quantity"=u16 16 ("number of coils"), "starting address"=u16 2500, "MB session in"=w259) -> ("error out"=w234:errorcluster, "Coils"=w255:bool[], "MB session out"=w235:refnum<class "MB_Master.lvclass">)  [unwired: 5 in]
            n162 = Index Array(array=w254) -> (element #1=→"X0":bool, element #2=→"X1":bool, element #3=→"X2":bool, element #4=→"X3":bool, element #5=→"X4":bool, element #6=w220:bool, element #7=→"X6":bool, element #8=→"X7":bool, element #9=→"X8":bool, element #10=→"X9":bool, element #11=→"X10":bool)  [unwired: 11 in]
            "X5" <- w220
            n163 = global write "采配水全局变量.vi" "关门信号"(w220) -> ()
            n164 = global write "采配水全局变量.vi" "报警簇"(w255) -> ()
          }
          frame "读参数" {
            n165 = call <vilib>:"Read Holding Registers.vi"("error in (no error)"=w305, "quantity"=u16 20 ("number of holding registers"), "starting address"=u16 100, "MB session in"=w306) -> ("error out"=w300:errorcluster, "Registers"=w302:u16[], "MB session out"=w301:refnum<class "MB_Master.lvclass">)  [unwired: 5 in]
            n166 = Array To Cluster(array=w302) -> (cluster=w284:T17)
            n167 = global write "采配水全局变量.vi" "参数设置"(w284) -> ()
            n168 = Unbundle(w284) -> ("Registers[0]"=→"R100":u16, "Registers[1]"=→"R101":u16, "Registers[2]"=→"R102":u16, "Registers[3]"=→"R103":u16, "Registers[4]"=→"R104":u16, "Registers[5]"=→"R105":u16, "Registers[6]"=→"R106":u16, "Registers[7]"=→"R107":u16, "Registers[8]"=→"R108":u16, "Registers[9]"=→"R109":u16, "Registers[10]"=w289:u16, "Registers[11]"=→"R111":u16, "Registers[12]"=→"R112":u16, "Registers[13]"=→"R113":u16, "Registers[18]"=→"R118":u16)  [unwired: 19 out]
            n169 = local write "潜水泵工作模式"(w289) -> ()
          }
          frame "多个写入" {
            n170 = Unbundle By Name(w312) -> ("数据"=w311:variant)
            n171 = Variant To Data(type=T12 {"starting address"=0, "holding register values"=[]}, Variant=w311) -> (data=w309:T12)  [unwired: 1 in, 1 out]
            n172 = Unbundle By Name(w309) -> ("starting address"=w308:u16, "holding register values"=w307:u16[])
            n173 = call <vilib>:"Write Multiple Registers.vi"("error in (no error)"=w315, "values"=w307, "starting address"=w308, "MB session in"=w316) -> ("error out"=w314:errorcluster, "MB session out"=w313:refnum<class "MB_Master.lvclass">)  [unwired: 6 in]
          }
          frame "单个写入" {
            n174 = Unbundle By Name(w322) -> ("数据"=w321:variant)
            n175 = Variant To Data(type=T13 {"starting address"=0, "holding register value"=0}, Variant=w321) -> (data=w319:T13)  [unwired: 1 in, 1 out]
            n176 = Unbundle By Name(w319) -> ("starting address"=w318:u16, "holding register value"=w317:u16)
            n177 = call <vilib>:"Write Single Register.vi"("error in (no error)"=w325, "value"=w317, "address"=w318, "MB session in"=w326) -> ("error out"=w324:errorcluster, "MB session out"=w323:refnum<class "MB_Master.lvclass">)  [unwired: 6 in]
          }
          frame "线圈写入" {
            n178 = Unbundle By Name(w332) -> ("数据"=w331:variant)
            n179 = Variant To Data(type=T14 {"starting address"=0, "coil values"=[]}, Variant=w331) -> (data=w329:T14)  [unwired: 1 in, 1 out]
            n180 = Unbundle By Name(w329) -> ("starting address"=w328:u16, "coil values"=w327:bool[])
            n181 = call <vilib>:"Write Multiple Coils.vi"("error in (no error)"=w335, "values"=w327, "starting address"=w328, "MB session in"=w336) -> ("error out"=w334:errorcluster, "MB session out"=w333:refnum<class "MB_Master.lvclass">)  [unwired: 6 in]
          }
          frame "shutdown" {
            n182 = call <vilib>:"Write Single Register.vi"("error in (no error)"=w343, "value"=u16 0, "address"=u16 4047, "MB session in"=w345) -> ("error out"=w344:errorcluster, "MB session out"=w342:refnum<class "MB_Master.lvclass">)  [unwired: 6 in]
            n183 = call-dynamic "Close Session.vi"("error in (no error)"=w344, "MB session in"=w342) -> ("error out"=w338:errorcluster)  [unwired: 9 in]
            n184 = call <vilib>:"Clear Errors.vi"("error in (no error)"=w338) -> ("error out"=w339:errorcluster)  [unwired: 5 in, 1 out]
            n185 = call "调用WinProladder.vi"("错误输入（无错误）"=w339) -> ("错误输出"=w337:errorcluster)  [unwired: 10 in]
          }
        }
      }
      frame Error {
        n186 = Unbundle By Name(w350) -> ("code"=w352:i32)
        n187 = case shown="-1073807343" w352 {
          tunnel: w351 -> [w354 w358]
          tunnel: w350 -> [w353 w360]
          tunnel: [w353 w359] -> w348
          tunnel: [w354 w358] -> w349
          tunnel: w346 -> [_ w357]
          frame Default {
          }
          frame -1073807343 {
            n188 = Flush Queue(queue=w357) -> (queue out=w356:refnum<queue>)  [unwired: 1 in, 2 out]
            n189 = call-dynamic "Close Session.vi"("error in (no error)"=w360, "MB session in"=w358) -> ("error out"=w359:errorcluster)  [unwired: 9 in]
            n190 = disable-structure shown="禁用" {
              disable-tunnel: w356 -> [w361 _]
              frame Disabled {
                n191 = Enqueue Element At Opposite End(queue=w361, element=cluster{"命令":string, "数据":variant} {"命令"="init", "数据"=variant} ("元素")) -> ()  [unwired: 2 in, 3 out]
              }
              frame Enabled {
              }
            }
            n192 = Wait (ms)(milliseconds to wait=u32 2000 ("等待时间（毫秒）")) -> ()  [unwired: 1 out]
          }
        }
        n193 = call <vilib>:"Clear Errors.vi"("error in (no error)"=w348) -> ("error out"=w347:errorcluster)  [unwired: 5 in, 1 out]
      }
    }
    n194 = Unbundle By Name(w186) -> ("status"=→"通讯故障":bool)
  }
  n195 = property on="多列列表框" class="MCListbox (严格)"("ItemNames"=string[][] [["待机"], ["初始化"], ["外部管路润洗"], ["内部管路润洗"], ["采样"], ["沉淀"], ["配水"], ["外部管路反冲洗"], ["内部管路反冲洗"], ["采样池储水"], ["结束"]] ("项名")) -> ()  [unwired: 2 in, 2 out]
  n196 = call-dynamic "Close Session.vi"("error in (no error)"=w8, "MB session in"=w7) -> ()  [unwired: 9 in, 1 out]
